vi "runConj.vi"() -> ()   [LabVIEW 2018]
uses:
  Daemon/RecipeEditor/Ctl/MSEditorParam updConj.ctl
panel:
  in  "Boolean":bool=TRUE
  in  "Freq":ext
  out "RfCyc_out":u64
  out "chaseCyc":u64
  out "Not Conj?":bool
  out "LastConj":bool
  in  "changeData":bool
  in  "update":bool
  in  "IniCycle":u64
  in  "Reset":bool
  in  "timeout in ms (-1)":i32=500
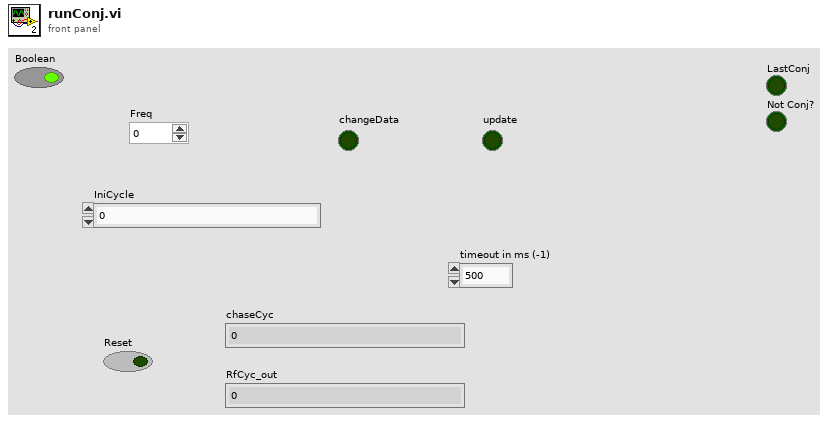
[diagram p1: front panel]
types:
  T1 = cluster{"Conj.InitCyc*2^32":u32, "ConjSize-1":u8, "ConjArr":cluster{"Ratio*2^15":u16, "CycleDiff":u64}[], "Mode":bool}
  T2 = typedef "MSEditorParam updConj.ctl" = cluster{"iniPhase":u32, "conjLen":ext[], "phaseDiff":u64[], "fixedLen":bool}
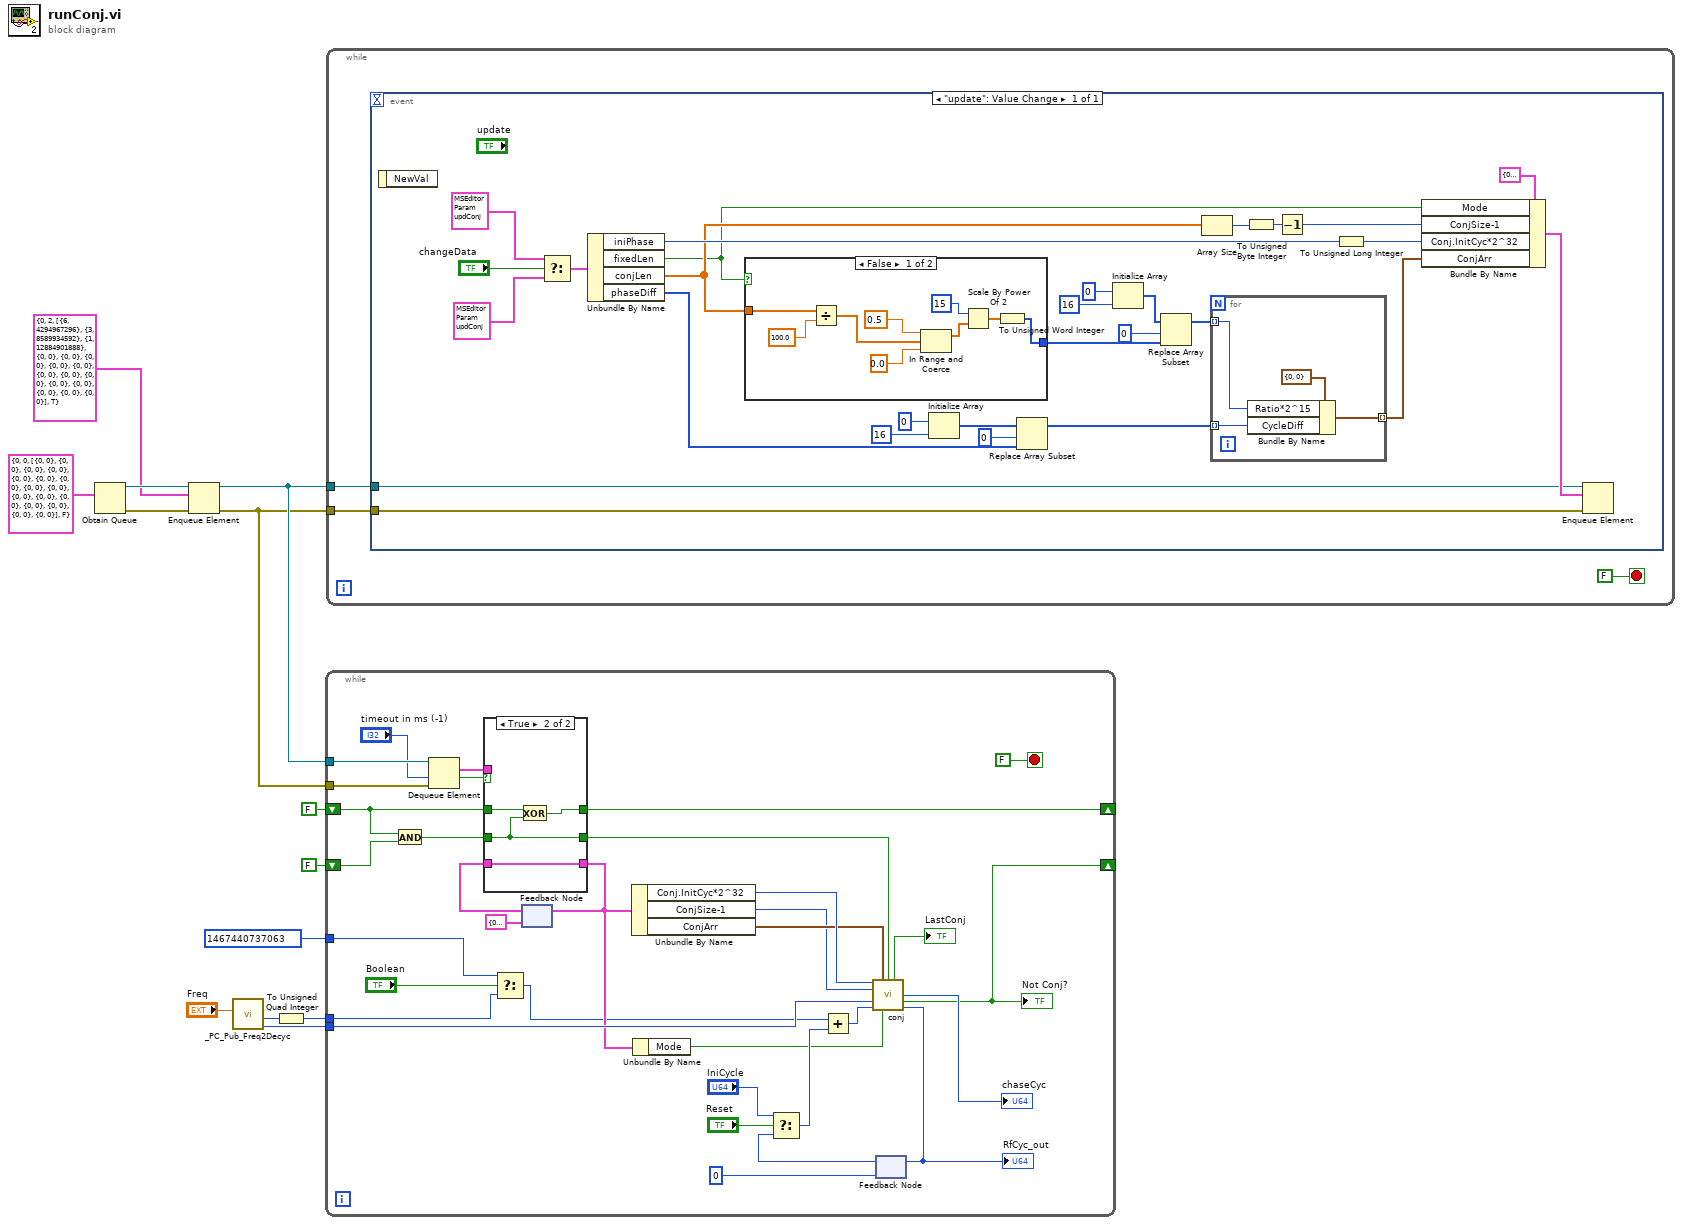
[diagram p0: block diagram]
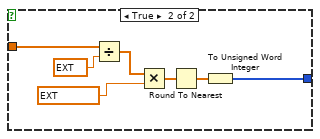
[diagram p2: hidden frame]
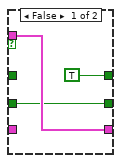
[diagram p3: hidden frame]
diagram:
  n1 = Obtain Queue(element data type=T1 {"Conj.InitCyc*2^32"=0, "ConjSize-1"=0, "ConjArr"=[{"Ratio*2^15"=0, "CycleDiff"=0}, {"Ratio*2^15"=0, "CycleDiff"=0}, {"Ratio*2^15"=0, "CycleDiff"=0}, {"Ratio*2^15"=0, "CycleDiff"=0}, {"Ratio*2^15"=0, "CycleDiff"=0}, {"Ratio*2^15"=0, "CycleDiff"=0}, {"Ratio*2^15"=0, "CycleDiff"=0}, {"Ratio*2^15"=0, "CycleDiff"=0}, {"Ratio*2^15"=0, "CycleDiff"=0}, {"Ratio*2^15"=0, "CycleDiff"=0}, {"Ratio*2^15"=0, "CycleDiff"=0}, {"Ratio*2^15"=0, "CycleDiff"=0}, {"Ratio*2^15"=0, "CycleDiff"=0}, {"Ratio*2^15"=0, "CycleDiff"=0}, {"Ratio*2^15"=0, "CycleDiff"=0}, {"Ratio*2^15"=0, "CycleDiff"=0}], "Mode"=FALSE}) -> (queue out=w8:refnum<queue>, error out=w7:errorcluster)  [unwired: 4 in, 1 out]
  n2 = Enqueue Element(queue=w8, element=T1 {"Conj.InitCyc*2^32"=0, "ConjSize-1"=2, "ConjArr"=[{"Ratio*2^15"=6, "CycleDiff"=4294967296}, {"Ratio*2^15"=3, "CycleDiff"=8589934592}, {"Ratio*2^15"=1, "CycleDiff"=12884901888}, {"Ratio*2^15"=0, "CycleDiff"=0}, {"Ratio*2^15"=0, "CycleDiff"=0}, {"Ratio*2^15"=0, "CycleDiff"=0}, {"Ratio*2^15"=0, "CycleDiff"=0}, {"Ratio*2^15"=0, "CycleDiff"=0}, {"Ratio*2^15"=0, "CycleDiff"=0}, {"Ratio*2^15"=0, "CycleDiff"=0}, {"Ratio*2^15"=0, "CycleDiff"=0}, {"Ratio*2^15"=0, "CycleDiff"=0}, {"Ratio*2^15"=0, "CycleDiff"=0}, {"Ratio*2^15"=0, "CycleDiff"=0}, {"Ratio*2^15"=0, "CycleDiff"=0}, {"Ratio*2^15"=0, "CycleDiff"=0}], "Mode"=TRUE} ("output cluster"), error in (no error)=w7) -> (queue out=w5:refnum<queue>, error out=w4:errorcluster)  [unwired: 1 in, 1 out]
  n3 = call "_PC_Pub_Freq2Decyc.vi"("Freq"="Freq") -> ("(1/Decyc)*2^8"=w13:u32, "Decyc*2^32"=w12:u32)  [unwired: 4 in, 3 out]
  n4 = To Unsigned Quad Integer(1:w12) -> (0:w11:u64)
  n5 = while {
    tunnel: w5 -> [w43]
    tunnel: w4 -> [w42]
    tunnel: w13 -> [w40]
    tunnel: w11 -> [w17]
    shift-right: [w29] -> _
    shift-left: FALSE ("Not Conj?") -> [w28]
    shift-right: [w24] -> _
    shift-left: FALSE -> [w21]
    tunnel: u64 1467440737063 ("t") -> [w14]
    stop <- FALSE stop-if-true
    n6 = And(x=w21, y=w28) -> (x .and. y?=w25:bool)
    n7 = Dequeue Element(queue=w43, timeout in ms (-1)="timeout in ms (-1)", error in (no error)=w42) -> (element=w26:T1, timed out?=w27:bool)  [unwired: 2 out]
    n8 = Select(t=w14, s="Boolean", f=w17) -> (s? t:f=w16:u64)
    n9 = feedback #1(T1 {"Conj.InitCyc*2^32"=0, "ConjSize-1"=0, "ConjArr"=[{"Ratio*2^15"=0, "CycleDiff"=0}, {"Ratio*2^15"=0, "CycleDiff"=0}, {"Ratio*2^15"=0, "CycleDiff"=0}, {"Ratio*2^15"=0, "CycleDiff"=0}, {"Ratio*2^15"=0, "CycleDiff"=0}, {"Ratio*2^15"=0, "CycleDiff"=0}, {"Ratio*2^15"=0, "CycleDiff"=0}, {"Ratio*2^15"=0, "CycleDiff"=0}, {"Ratio*2^15"=0, "CycleDiff"=0}, {"Ratio*2^15"=0, "CycleDiff"=0}, {"Ratio*2^15"=0, "CycleDiff"=0}, {"Ratio*2^15"=0, "CycleDiff"=0}, {"Ratio*2^15"=0, "CycleDiff"=0}, {"Ratio*2^15"=0, "CycleDiff"=0}, {"Ratio*2^15"=0, "CycleDiff"=0}, {"Ratio*2^15"=0, "CycleDiff"=0}], "Mode"=FALSE}) -> (w23:T1)
    n10 = case shown="True" w27 {
      tunnel: w26 -> [w48 _]
      tunnel: w25 -> [w47 w51]
      tunnel: [TRUE w50] -> w24
      tunnel: [w48 w53] -> w19
      tunnel: w23 -> [_ w53]
      tunnel: [w47 w51] -> w22
      tunnel: w21 -> [_ w52]
      frame False {
      }
      frame True {
        n11 = Exclusive Or(1:w51, 2:w52) -> (0:w50:bool)
      }
    }
    n12 = feedback-in #1(w19) -> ()
    n13 = Unbundle By Name(w19) -> ("Conj.InitCyc*2^32"=w34:u32, "ConjSize-1"=w32:u8, "ConjArr"=w33:cluster{"Ratio*2^15":u16, "CycleDiff":u64}[])
    n14 = Unbundle By Name(w19) -> ("Mode"=w18:bool)
    n15 = feedback #2(u64 0 ("RfCyc_out")) -> (w37:u64)
    n16 = Select(t="IniCycle", s="Reset", f=w37) -> (s? t:f=w36:u64)
    n17 = Add(x=w16, y=w36) -> (x+y=w45:u64)
    n18 = call "conj.vi"("Conj.InitCyc*2^32"=w34, "ConjArr"=w33, "Init_strobe"=w22, "ConjSize-1"=w32, "1/DeCyc*2^8"=w40, "RfCyc_in"=w45, "Mode"=w18) -> ("LastConj"=→"LastConj":bool, "chaseCyc"=→"chaseCyc":u64, "Not Conj?"=w29:bool, "RfCyc_out"=w46:u64)  [unwired: 3 in, 2 out]
    "Not Conj?" <- w29
    "RfCyc_out" <- w46
    n19 = feedback-in #2(w46) -> ()
  }
  n20 = while {
    tunnel: w5 -> [w56]
    tunnel: w4 -> [w55]
    stop <- FALSE stop-if-true
    n21 = event shown="[0] \"update\": Value Change" {
      selector: _ -> [_]
      dyn-events: _ -> [_]
      timeout: _ -> [_]
      tunnel: w56 -> [w62]
      tunnel: w55 -> [w61]
      event "update": Value Change {
        n22 = event-data() -> ()  [unwired: 1 in, 1 out]
        n23 = Select(t=T2 {"iniPhase"=0, "conjLen"=[0.00015, 0.000075, 0.000025], "phaseDiff"=[4294967296, 8589934592, 12884901888], "fixedLen"=TRUE} ("ParamValueType"), s="changeData", f=T2 {"iniPhase"=2147483648, "conjLen"=[0.0, 0.0], "phaseDiff"=[2147483648, 2147483648], "fixedLen"=FALSE} ("ParamValueType")) -> (s? t:f=w57:T2)
        n24 = Unbundle By Name(w57) -> ("iniPhase"=w74:u32, "fixedLen"=w69:bool, "conjLen"=w72:ext[], "phaseDiff"=w73:u64[])
        n25 = case shown="False" w69 {
          tunnel: w72 -> [w90 w104]
          tunnel: [w89 w98] -> w71
          frame False {
            n26 = Divide(x=w90, y=100.0) -> (x/y=w97:ext[])
            n27 = In Range and Coerce(upper limit=0.5, x=w97, lower limit=0.0) -> (coerced(x)=w94:ext[])  [unwired: 1 out]
            n28 = Scale By Power Of 2(n=i16 15, x=w94) -> (x*2^n=w92:ext[])
            n29 = To Unsigned Word Integer(number=w92) -> (unsigned 16bit integer=w89:u16[])
          }
          frame True {
            n30 = Divide(x=w104, y=ext 1000.0) -> (x/y=w101:ext[])
            n31 = Multiply(x=w101, y=ext 40000000.0) -> (x*y=w100:ext[])
            n32 = Round To Nearest(number=w100) -> (nearest integer value=w99:ext[])
            n33 = To Unsigned Word Integer(number=w99) -> (unsigned 16bit integer=w98:u16[])
          }
        }
        n34 = Initialize Array(u64 0, 16 ("dimension size")) -> (w81:u64[])
        n35 = Replace Array Subset(array=w81, new element=w73, index=0) -> (w65:u64[])
        n36 = Initialize Array(u16 0, 16 ("dimension size")) -> (w79:u16[])
        n37 = Replace Array Subset(array=w79, new element=w71, index=0) -> (w66:u16[])
        n38 = Array Size(array=w72) -> (size(s)=w84:i32)
        n39 = for {
          tunnel: w66 -> [w88] mode=indexing
          tunnel: w65 -> [w87] mode=indexing
          tunnel: [w86] -> w64 mode=indexing
          n40 = Bundle By Name(cluster=cluster{"Ratio*2^15":u16, "CycleDiff":u64} {"Ratio*2^15"=0, "CycleDiff"=0} ("Cluster"), "Ratio*2^15"=w88, "CycleDiff"=w87) -> (w86:cluster{"Ratio*2^15":u16, "CycleDiff":u64})
        }
        n41 = To Unsigned Byte Integer(number=w84) -> (unsigned 8bit integer=w75:u8)
        n42 = Decrement(x=w75) -> (x-1=w68:u8)
        n43 = To Unsigned Long Integer(number=w74) -> (unsigned 32bit integer=w67:u32)
        n44 = Bundle By Name(cluster=T1 {"Conj.InitCyc*2^32"=0, "ConjSize-1"=0, "ConjArr"=[{"Ratio*2^15"=0, "CycleDiff"=0}, {"Ratio*2^15"=0, "CycleDiff"=0}, {"Ratio*2^15"=0, "CycleDiff"=0}, {"Ratio*2^15"=0, "CycleDiff"=0}, {"Ratio*2^15"=0, "CycleDiff"=0}, {"Ratio*2^15"=0, "CycleDiff"=0}, {"Ratio*2^15"=0, "CycleDiff"=0}, {"Ratio*2^15"=0, "CycleDiff"=0}, {"Ratio*2^15"=0, "CycleDiff"=0}, {"Ratio*2^15"=0, "CycleDiff"=0}, {"Ratio*2^15"=0, "CycleDiff"=0}, {"Ratio*2^15"=0, "CycleDiff"=0}, {"Ratio*2^15"=0, "CycleDiff"=0}, {"Ratio*2^15"=0, "CycleDiff"=0}, {"Ratio*2^15"=0, "CycleDiff"=0}, {"Ratio*2^15"=0, "CycleDiff"=0}], "Mode"=FALSE}, "Mode"=w69, "ConjSize-1"=w68, "Conj.InitCyc*2^32"=w67, "ConjArr"=w64) -> (w63:T1)
        n45 = Enqueue Element(queue=w62, element=w63, error in (no error)=w61) -> ()  [unwired: 1 in, 3 out]
      }
    }
  }
